vi "Write Element of VI refs.vi"(8 "error in (no error)":errorcluster, 9 "vi reference":refnum<vi>, 10 "index":i32=-1, 11 "Control in":refnum<class "Control-Server.lvclass">) -> (0 "error out":errorcluster, 3 "Control out":refnum<class "Control-Server.lvclass">)   [LabVIEW 2019, in "Control-Server.lvclass"]
uses:
  Control-Server.lvclass
  Control-Server.lvclass/Control-Server.ctl
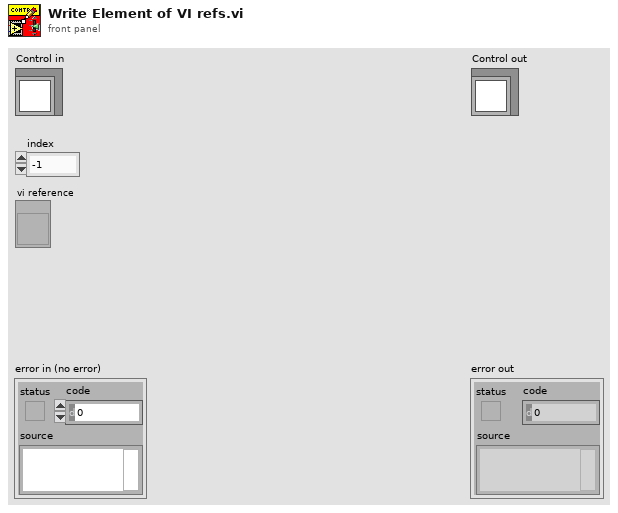
[diagram p1: front panel]
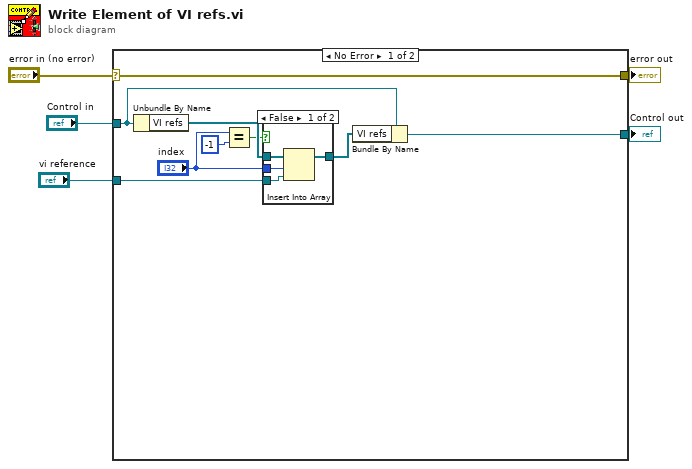
[diagram p0: block diagram]
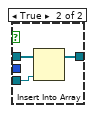
[diagram p2: hidden frame]
diagram:
  n1 = case shown="No Error" "error in (no error)" {
    selector: "error in (no error)" -> [w14 w22]
    tunnel: [w14 w22] -> w4
    tunnel: [w13 w23] -> w2
    tunnel: "Control in" -> [w12 w23]
    tunnel: "vi reference" -> [w10 _]
    frame No Error {
      n2 = Unbundle By Name(w12) -> ("VI refs"=w9:refnum<vi>[])
      n3 = Equal?(x="index", y=-1) -> (x = y?=w6:bool)
      n4 = case shown="False" w6 {
        tunnel: w10 -> [w17 w21]
        tunnel: w9 -> [w15 w20]
        tunnel: [w16 w19] -> w8
        tunnel: "index" -> [w18 _]
        frame False {
          n5 = Insert Into Array(array=w15, index=w18, new element=w17) -> (w16:refnum<vi>[])
        }
        frame True {
          n6 = Insert Into Array(array=w20, new element=w21) -> (w19:refnum<vi>[])  [unwired: 1 in]
        }
      }
      n7 = Bundle By Name(cluster=w12, "VI refs"=w8) -> (w13:refnum<class "Control-Server.lvclass">)
    }
    frame Error {
    }
  }
  "error out" <- w4
  "Control out" <- w2
